vi "GUI_StagingDischarge.vi"() -> ()   [LabVIEW 2013]
uses:
  shared programs/GUI_Template/GUI_master/tcp new data cluster.ctl
  Device Driver/shared/stop FGV control.ctl
panel:
  in  "enable.hv 2::1":bool
  in  "enable.hv 1::1":bool
  in  "voltage.hv 2::1":dbl caption="Output 2"
  in  "voltage.hv 1::1":dbl
  out "device status::1":string="Initialized" caption="Status"
  in  "stop":bool
  in  "GUIdevice 1":string="StagingDischargeHV"
  # "DAQ PAD USER INTERFACE"
  # "Voltage (kV)"
  # "Enable"
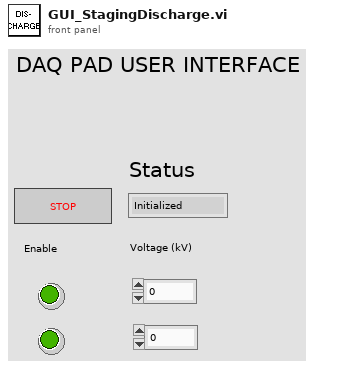
[diagram p1: front panel]
types:
  T1 = typedef "stop FGV control.ctl" = enum16{"Clear", "Write", "Read"}
  T2 = typedef "tcp new data cluster.ctl" = cluster{"EventEnum":enum16{"new data", "connection status update"}, "Device name":string}
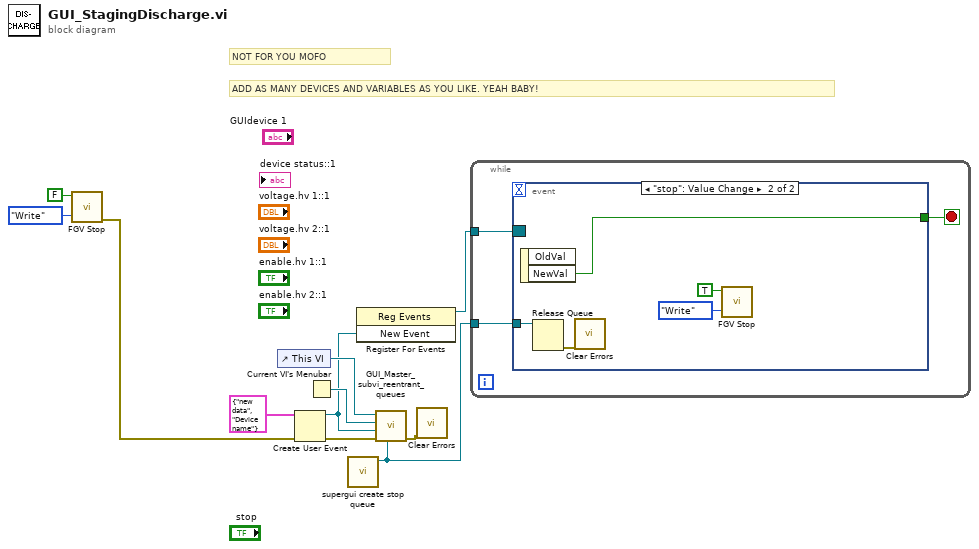
[diagram p0: block diagram]
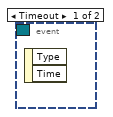
[diagram p2: hidden frame]
diagram:
  # "ADD AS MANY DEVICES AND VARIABLES AS YOU LIKE. YEAH BABY!"
  # "NOT FOR YOU MOFO"
  n1 = call "FGV Stop.vi"("Function"=stop_FGV_control."Write", "stop"=FALSE) -> ("error out"=w2:errorcluster)  [unwired: 8 in, 1 out]
  n2 = control-ref of="This VI"() -> (w11:refnum<vi>)
  n3 = Create User Event(user event datatype=T2 {"EventEnum"=enum."new data", "Device name"="Device name"} ("New Event"), error in=w2) -> (user event=w6:refnum<user-event>, error out=w8:errorcluster)
  n4 = Current VI's Menubar() -> (w10:refnum<k9>)
  n5 = call "supergui create stop queue.vi"() -> ("STOP Queue out"=w1:refnum<queue>)  [unwired: 11 in]
  n6 = register-events(w6) -> (reference out=w5:refnum<event-registration>)  [unwired: 2 in, 1 out]
  n7 = call "GUI_Master_subvi_reentrant_queues.vi"("STOP Queue in"=w1, "error in (no error)"=w8, "tcp data event"=w6, "Caller menu reference"=w10, "Caller VI ref"=w11) -> ("error out"=w7:errorcluster)  [unwired: 6 in]
  n8 = call <vilib>:"Clear Errors.vi"("error in (no error)"=w7) -> ()  [unwired: 6 in, 1 out]
  n9 = while {
    tunnel: w5 -> [w14]
    tunnel: w1 -> [w12]
    stop <- w13 stop-if-true
    n10 = event shown="[1] \"stop\": Value Change" {
      selector: w14 -> [_ _]
      dyn-events: _ -> [_ _]
      timeout: _ -> [_ _]
      tunnel: [_ w19] -> w13
      tunnel: w12 -> [_ w16]
      event Timeout {
        n11 = event-data() -> ()  [unwired: 1 in, 2 out]
      }
      event "stop": Value Change {
        n12 = event-data() -> ("NewVal"=w19:bool)  [unwired: 1 in, 1 out]
        n13 = Release Queue(queue=w16) -> (error out=w15:errorcluster)  [unwired: 2 in, 2 out]
        n14 = call <vilib>:"Clear Errors.vi"("error in (no error)"=w15) -> ()  [unwired: 6 in, 1 out]
        n15 = call "FGV Stop.vi"("Function"=stop_FGV_control."Write", "stop"=TRUE) -> ()  [unwired: 8 in, 2 out]
      }
    }
  }
